vi "Check Manager Queue.vi"(8 "error in (no error)":errorcluster, 11 "Channel Manager in":refnum<class "Channel Manager.lvclass">) -> (0 "error out":errorcluster, 1 "queue ref invalid":bool, 3 "Channel Manager out":refnum<class "Channel Manager.lvclass">)   [LabVIEW 2024, in "Channel Manager.lvclass"]
uses:
  Channel Manager.lvclass
  Channel Manager.lvclass/Channel Manager.ctl
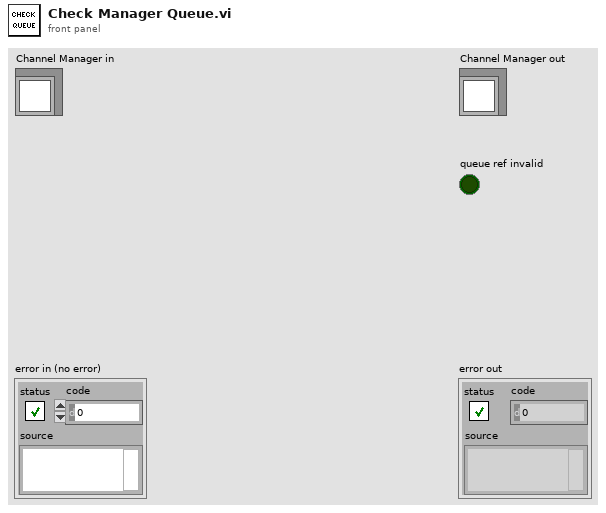
[diagram p1: front panel]
types:
  T1 = typedef "AIM ARINC 429 Hardware API.lvlib/Channel Status.ctl" = enum16{"Uninitialized", "Idle", "Active"}
  T2 = map{cluster{"board handle":u8, "channel number":u8}, cluster{"count":u32, "status":T1}}
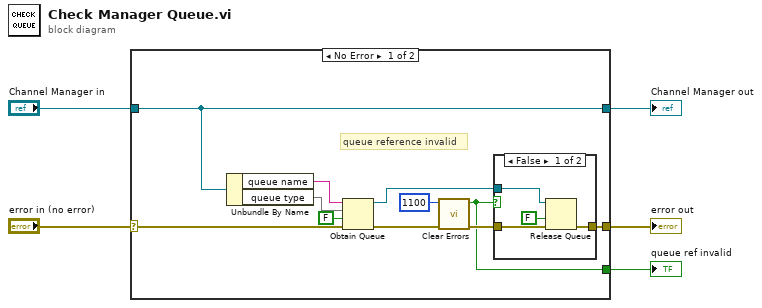
[diagram p0: block diagram]
diagram:
  n1 = case shown="No Error" "error in (no error)" {
    selector: "error in (no error)" -> [w13 w23]
    tunnel: [w7 w23] -> w4
    tunnel: [w14 w22] -> w2
    tunnel: "Channel Manager in" -> [w14 w22]
    tunnel: [w6 _] -> w1
    frame No Error {
      # "queue reference invalid"
      n2 = Unbundle By Name(w14) -> ("queue name"=w16:string, "queue type"=w15:T2)
      n3 = Obtain Queue(name (unnamed)=w16, element data type=w15, create if not found? (T)=FALSE, error in (no error)=w13) -> (queue out=w8:refnum<queue>, error out=w11:errorcluster)  [unwired: 1 in, 1 out]
      n4 = call <vilib>:"Clear Errors.vi"("error in (no error)"=w11, "specific error code to clear (0: all)"=1100) -> ("error out"=w9:errorcluster, "specific error cleared?"=w6:bool)  [unwired: 4 in]
      n5 = case shown="False" w6 {
        tunnel: w9 -> [w20 w21]
        tunnel: w8 -> [w19 _]
        tunnel: [w17 w21] -> w7
        frame False {
          n6 = Release Queue(queue=w19, force destroy? (F)=FALSE, error in (no error)=w20) -> (error out=w17:errorcluster)  [unwired: 2 out]
        }
        frame True {
        }
      }
    }
    frame Error {
    }
  }
  "error out" <- w4
  "Channel Manager out" <- w2
  "queue ref invalid" <- w1
